vi "getWavelength_v60.vi"() -> ()   [LabVIEW 2012]
uses:
  x32/CLDevIFace.dll
panel:
  in  "stop":bool
  in  "OK Button":bool
  out "Wavelength":dbl
  in  "CommPort":dbl caption="Comm Port #"
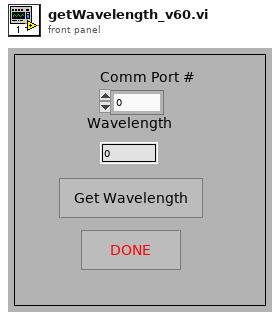
[diagram p1: front panel]
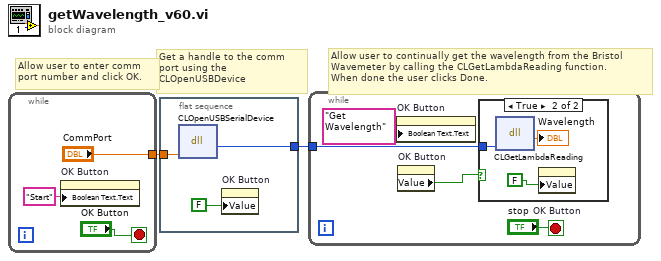
[diagram p0: block diagram]
diagram:
  # "Allow user to continually get the wavelength from the Bristol\nWavemeter by calling the CLGetLambdaReading function.  \nWhen done the user clicks Done."
  # "Get a handle to the comm\nport using the CLOpenUSBDevice"
  # "Allow user to enter comm \nport number and click OK."
  n1 = while {
    tunnel: ["CommPort"] -> w2
    stop <- "OK Button" stop-if-true
    n2 = property on="OK Button" class="Bool (strict)"("Boolean Text.Text"="Start") -> ()  [unwired: 2 in, 2 out]
  }
  n3 = flat-sequence {
    tunnel: w2 -> [w8]
    tunnel: [w7] -> w1
    frame #0 {
      n4 = dll-call lib="C:/Users/Lab/Desktop/Bristol wavemeter 621/00424-2-00 621 customer CD/Programming Interface/x32/CLDevIface.dll" fn="CLOpenUSBSerialDevice"("commPort"=w8) -> (w7:i32)  [unwired: 4 in, 2 out]
      n5 = property on="OK Button" class="Bool (strict)"("Value"=FALSE) -> ()  [unwired: 2 in, 2 out]
    }
  }
  n6 = while {
    tunnel: w1 -> [w12]
    stop <- "stop" stop-if-true
    n7 = property on="OK Button" class="Bool (strict)"("Boolean Text.Text"="Get Wavelength") -> ()  [unwired: 2 in, 2 out]
    n8 = property on="OK Button" class="Bool (strict)"() -> ("Value"=w9:bool)  [unwired: 2 in, 2 out]
    n9 = case shown="True" w9 {
      tunnel: w12 -> [_ w15]
      frame False {
      }
      frame True {
        n10 = dll-call lib="C:/Users/Lab/Desktop/Bristol wavemeter 621/00424-2-00 621 customer CD/Programming Interface/x32/CLDevIface.dll" fn="CLGetLambdaReading"("devHandle"=w15) -> (→"Wavelength":dbl)  [unwired: 4 in, 2 out]
        n11 = property on="OK Button" class="Bool (strict)"("Value"=FALSE) -> ()  [unwired: 2 in, 2 out]
      }
    }
  }
